vi "xiC - IMAQ - GetPRMToSave.vi"(8 "error in (no error)":errorcluster, 11 "Attributes In":T2) -> (0 "error out":errorcluster, 1 "PRM[] to Save":T1[](array[typedef]), 3 "Attributes Out":T2)   [LabVIEW 2015]
uses:
  xiCamLib/xiCam/PRM/PRM/PRM_v2.ctl
  xiC - IMAQ - Attributes.ctl
  C:/GIT/Cameras3.x/Integrations/Labview/xiLib/xiLIB_32bit/xiLIB/xiCamLib/API/x86/xiApi.NET.dll
  xiLIB_32bit/xiLIB/xiCamLib/API/x86/xiApi.NET.dll
  xiC - IMAQ - TreeDisplayType.ctl
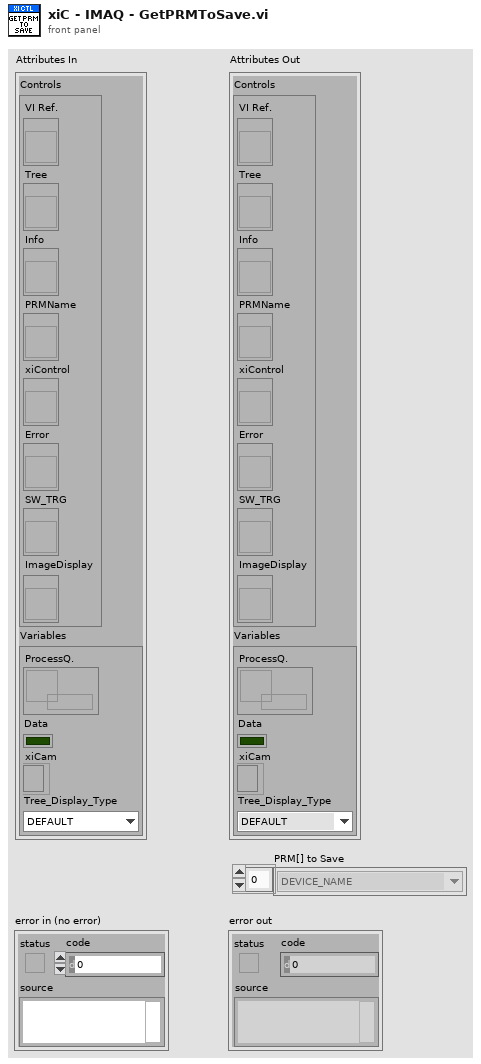
[diagram p1: front panel]
types:
  T1 = typedef "PRM_v2.ctl" = enum16{"ACQ_BUFFER_SIZE", "ACQ_FRAME_BURST_COUNT", "ACQ_TIMING_MODE", "ACQ_TRANSPORT_BUFFER_SIZE", "AE_MAX_LIMIT", "AEAG", "AEAG_LEVEL", "API_VERSION", "AG_MAX_LIMIT", "APPLY_CMS", "AUTO_BANDWIDTH_CALCULATION", "AUTO_WB", "AVAILABLE_BANDWIDTH", "AVAILABLE_BANDWIDTH_MAX", "AVAILABLE_BANDWIDTH_MIN", "BPC", "BUFFER_POLICY", "BUFFERS_QUEUE_SIZE", "CC_MATRIX_00", "CC_MATRIX_01", "CC_MATRIX_02", "CC_MATRIX_03", "CC_MATRIX_10", "CC_MATRIX_11", "CC_MATRIX_12", "CC_MATRIX_13", "CC_MATRIX_20", "CC_MATRIX_21", "CC_MATRIX_22", "CC_MATRIX_23", "CC_MATRIX_30", "CC_MATRIX_31", "CC_MATRIX_32", "CC_MATRIX_33", "CHIP_TEMP", "CMS", "COLOR_FILTER_ARRAY", "COOLING", "DEBOUNCE_EN", "DEBOUNCE_POL", "DEBOUNCE_T0", "DEBOUNCE_T1", "DEBUG_LEVEL", "DEFAULT_CC_MATRIX", "DEVICE_INSTANCE_PATH", "DEVICE_MODEL_ID", "DEVICE_NAME", "DEVICE_SN", "DEVICE_TYPE", "DEVICE_USER_ID", "DOWNSAMPLING", "DOWNSAMPLING_MAX", "DOWNSAMPLING_MIN", "DOWNSAMPLING_TYPE", "DRV_VERSION", "EXP_PRIORITY", "EXPOSURE", "EXPOSURE_DIRECT_UPDATE", "EXPOSURE_MAX", "EXPOSURE_MIN", "FFS_FILE_NAME", "FPGA1_VERSION", "FRAMERATE", "FRAMERATE_MAX", "FRAMERATE_MIN", "FREE_FFS_SIZE", "GAIN", "GAIN_DIRECT_UPDATE", "GAIN_MAX", "GAIN_MIN", "GAMMAC", "GAMMAY", "GPI_LEVEL", "GPI_MODE", "GPI_SELECTOR", "GPI_SELECTOR_MAX", "GPI_SELECTOR_MIN", "GPO_MODE", "GPO_SELECTOR", "GPO_SELECTOR_MAX", "GPO_SELECTOR_MIN", "HDR", "HDR_T1", "HDR_T2", "HEIGHT", "HEIGHT_MAX", "HEIGHT_MIN", "HOUSE_TEMP", "IMAGE_DATA_FORMAT", "IMAGE_IS_COLOR", "INPUT_CMS_PROFILE", "IS_COOLED", "IS_DEVICE_EXIST", "KNEEPOINT1", "KNEEPOINT2", "LED_MODE", "LED_SELECTOR", "LED_SELECTOR_MAX", "LED_SELECTOR_MIN", "LIMIT_BANDWIDTH", "LIMIT_BANDWIDTH_MAX", "LIMIT_BANDWIDTH_MIN", "LUT_EN", "LUT_INDEX", "LUT_INDEX_MAX", "LUT_INDEX_MIN", "LUT_VALUE", "LUT_VALUE_MAX", "LUT_VALUE_MIN", "MANUAL_WB", "MCU1_VERSION", "MCU2_VERSION", "OFFSET_X", "OFFSET_X_MAX", "OFFSET_X_MIN", "OFFSET_Y", "OFFSET_Y_MAX", "OFFSET_Y_MIN", "OUTPUT_CMS_PROFILE", "OUTPUT_DATA_BIT_DEPTH", "OUTPUT_DATA_PACKING", "READ_FILE_FFS", "RECENT_FRAME", "SENSOR_DATA_BIT_DEPTH", "SENSOR_MODE", "SENSOR_TAPS", "SHARPNESS", "SHUTTER_TYPE", "TARGET_TEMP", "TRG_DELAY", "TRG_SELECTOR", "TRG_SOFTWARE", "TRG_SOURCE", "USED_FFS_SIZE", "WB_KB", "WB_KG", "WB_KR", "WIDTH", "WIDTH_MAX", "WIDTH_MIN", "WRITE_FILE_FFS", "ACQ_BUFFER_SIZE_UNIT", "ACQ_TRANSPORT_BUFFER_COMMIT", "AEAG_ROI_HEIGHT", "AEAG_ROI_OFFSET_X", "AEAG_ROU_OFFSET_Y", "AEAG_ROI_WIDTH", "API_CONTEXT_LIST", "BINNING_HORIZONTAL", "BINNING_SELECTOR", "BINNING_VERTICAL", "COLUMN_FPN_CORRECTION", "COUNTER_SELECTOR", "COUNTER_VALUE", "DECIMATION_HORIZONTAL", "DECIMATION_SELECTOR", "DECIMATION_VERTICAL", "DEVICE_ID", "DEVICE_LOCATION_PATH", "DEVICE_MANIFEST", "DEVICE_RESET", "DEVICE_SENS_SN", "EXPOSURE_BURST_COUNT", "FFS_ACCESS_KEY", "GAIN_SELECTOR", "HW_REVISION", "IMAGE_BLACK_LEVEL", "IMAGE_DATA_BIT_DEPTH", "IMAGE_DATA_FORMAT_RGB32_ALPHA", "IMAGE_PAYLOAD_SIZE", "LENS_APERTURE_VALUE", "LENS_FEATURE", "LENS_FEATURE_SELECTOR", "LENS_FOCAL_LENGTH", "LENS_FOCUS_DISTANCE", "LENS_FOCUS_MOVE", "LENS_FOCUS_MOVEMENT_VALUE", "LENS_MODE", "OUTPUT_DATA_PACKING_TYPE", "SENSOR_CLOCK_FREQ_HZ", "SENSOR_CLOCK_FREQ_INDEX", "SENSOR_FEATURE_SELECTOR", "SENSOR_FEATURE_VALUE", "SENSOR_OUTPUT_CHANNEL_COUNT", "TRANSPORT_PIXEL_FORMAT", "TS_RST_MODE", "TS_RST_SOURCE"}
  T2 = typedef "xiC - IMAQ - Attributes.ctl" = cluster{"Controls":cluster{"VI Ref.":refnum<vi>, "Tree":refnum<vi>, "Info":refnum<vi>, "PRMName":refnum<vi>, "xiControl":refnum<vi>, "Error":refnum<vi>, "SW_TRG":refnum<vi>, "ImageDisplay":refnum<vi>}, "Variables":cluster{"ProcessQ.":refnum<queue>, "Data":bool, "xiCam":refnum<k24>, "Tree_Display_Type":T3}}
  T3 = typedef "xiC - IMAQ - TreeDisplayType.ctl" = enum16{"DEFAULT", "HIDE_MAX_MIN"}
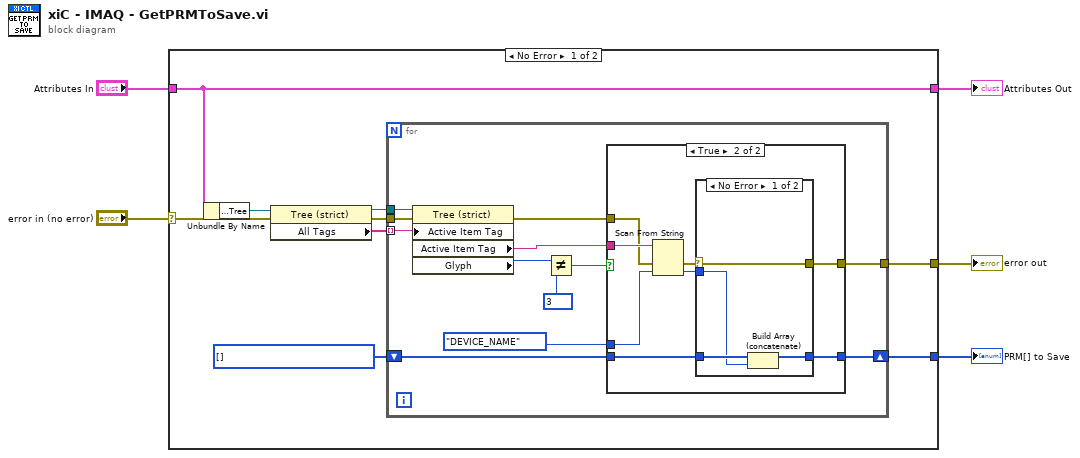
[diagram p0: block diagram]
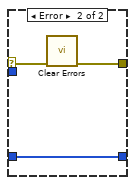
[diagram p3: hidden frame]
diagram:
  n1 = case shown="No Error" "error in (no error)" {
    selector: "error in (no error)" -> [w12 w45]
    tunnel: [w7 w45] -> w4
    tunnel: "Attributes In" -> [w13 w44]
    tunnel: [w13 w44] -> w2
    tunnel: [w6 _] -> w1
    frame No Error {
      w8 = T1[] [] items=["ACQ_BUFFER_SIZE", "ACQ_FRAME_BURST_COUNT", "ACQ_TIMING_MODE", "ACQ_TRANSPORT_BUFFER_SIZE", "AE_MAX_LIMIT", "AEAG", "AEAG_LEVEL", "API_VERSION", "AG_MAX_LIMIT", "APPLY_CMS", "AUTO_BANDWIDTH_CALCULATION", "AUTO_WB", "AVAILABLE_BANDWIDTH", "AVAILABLE_BANDWIDTH_MAX", "AVAILABLE_BANDWIDTH_MIN", "BPC", "BUFFER_POLICY", "BUFFERS_QUEUE_SIZE", "CC_MATRIX_00", "CC_MATRIX_01", "CC_MATRIX_02", "CC_MATRIX_03", "CC_MATRIX_10", "CC_MATRIX_11", "CC_MATRIX_12", "CC_MATRIX_13", "CC_MATRIX_20", "CC_MATRIX_21", "CC_MATRIX_22", "CC_MATRIX_23", "CC_MATRIX_30", "CC_MATRIX_31", "CC_MATRIX_32", "CC_MATRIX_33", "CHIP_TEMP", "CMS", "COLOR_FILTER_ARRAY", "COOLING", "DEBOUNCE_EN", "DEBOUNCE_POL", "DEBOUNCE_T0", "DEBOUNCE_T1", "DEBUG_LEVEL", "DEFAULT_CC_MATRIX", "DEVICE_INSTANCE_PATH", "DEVICE_MODEL_ID", "DEVICE_NAME", "DEVICE_SN", "DEVICE_TYPE", "DEVICE_USER_ID", "DOWNSAMPLING", "DOWNSAMPLING_MAX", "DOWNSAMPLING_MIN", "DOWNSAMPLING_TYPE", "DRV_VERSION", "EXP_PRIORITY", "EXPOSURE", "EXPOSURE_DIRECT_UPDATE", "EXPOSURE_MAX", "EXPOSURE_MIN", "FFS_FILE_NAME", "FPGA1_VERSION", "FRAMERATE", "FRAMERATE_MAX", "FRAMERATE_MIN", "FREE_FFS_SIZE", "GAIN", "GAIN_DIRECT_UPDATE", "GAIN_MAX", "GAIN_MIN", "GAMMAC", "GAMMAY", "GPI_LEVEL", "GPI_MODE", "GPI_SELECTOR", "GPI_SELECTOR_MAX", "GPI_SELECTOR_MIN", "GPO_MODE", "GPO_SELECTOR", "GPO_SELECTOR_MAX", "GPO_SELECTOR_MIN", "HDR", "HDR_T1", "HDR_T2", "HEIGHT", "HEIGHT_MAX", "HEIGHT_MIN", "HOUSE_TEMP", "IMAGE_DATA_FORMAT", "IMAGE_IS_COLOR", "INPUT_CMS_PROFILE", "IS_COOLED", "IS_DEVICE_EXIST", "KNEEPOINT1", "KNEEPOINT2", "LED_MODE", "LED_SELECTOR", "LED_SELECTOR_MAX", "LED_SELECTOR_MIN", "LIMIT_BANDWIDTH", "LIMIT_BANDWIDTH_MAX", "LIMIT_BANDWIDTH_MIN", "LUT_EN", "LUT_INDEX", "LUT_INDEX_MAX", "LUT_INDEX_MIN", "LUT_VALUE", "LUT_VALUE_MAX", "LUT_VALUE_MIN", "MANUAL_WB", "MCU1_VERSION", "MCU2_VERSION", "OFFSET_X", "OFFSET_X_MAX", "OFFSET_X_MIN", "OFFSET_Y", "OFFSET_Y_MAX", "OFFSET_Y_MIN", "OUTPUT_CMS_PROFILE", "OUTPUT_DATA_BIT_DEPTH", "OUTPUT_DATA_PACKING", "READ_FILE_FFS", "RECENT_FRAME", "SENSOR_DATA_BIT_DEPTH", "SENSOR_MODE", "SENSOR_TAPS", "SHARPNESS", "SHUTTER_TYPE", "TARGET_TEMP", "TRG_DELAY", "TRG_SELECTOR", "TRG_SOFTWARE", "TRG_SOURCE", "USED_FFS_SIZE", "WB_KB", "WB_KG", "WB_KR", "WIDTH", "WIDTH_MAX", "WIDTH_MIN", "WRITE_FILE_FFS", "ACQ_BUFFER_SIZE_UNIT", "ACQ_TRANSPORT_BUFFER_COMMIT", "AEAG_ROI_HEIGHT", "AEAG_ROI_OFFSET_X", "AEAG_ROU_OFFSET_Y", "AEAG_ROI_WIDTH", "API_CONTEXT_LIST", "BINNING_HORIZONTAL", "BINNING_SELECTOR", "BINNING_VERTICAL", "COLUMN_FPN_CORRECTION", "COUNTER_SELECTOR", "COUNTER_VALUE", "DECIMATION_HORIZONTAL", "DECIMATION_SELECTOR", "DECIMATION_VERTICAL", "DEVICE_ID", "DEVICE_LOCATION_PATH", "DEVICE_MANIFEST", "DEVICE_RESET", "DEVICE_SENS_SN", "EXPOSURE_BURST_COUNT", "FFS_ACCESS_KEY", "GAIN_SELECTOR", "HW_REVISION", "IMAGE_BLACK_LEVEL", "IMAGE_DATA_BIT_DEPTH", "IMAGE_DATA_FORMAT_RGB32_ALPHA", "IMAGE_PAYLOAD_SIZE", "LENS_APERTURE_VALUE", "LENS_FEATURE", "LENS_FEATURE_SELECTOR", "LENS_FOCAL_LENGTH", "LENS_FOCUS_DISTANCE", "LENS_FOCUS_MOVE", "LENS_FOCUS_MOVEMENT_VALUE", "LENS_MODE", "OUTPUT_DATA_PACKING_TYPE", "SENSOR_CLOCK_FREQ_HZ", "SENSOR_CLOCK_FREQ_INDEX", "SENSOR_FEATURE_SELECTOR", "SENSOR_FEATURE_VALUE", "SENSOR_OUTPUT_CHANNEL_COUNT", "TRANSPORT_PIXEL_FORMAT", "TS_RST_MODE", "TS_RST_SOURCE"]
      n2 = Unbundle By Name(w13) -> ("Controls.Tree"=w14:refnum<vi>)
      n3 = property class="Tree (strict)"(reference=w14, error in=w12) -> (reference out=w11:refnum<vi>, error out=w10:errorcluster, "All Tags"=w9:string[])
      n4 = for {
        tunnel: w11 -> [w26]
        tunnel: w10 -> [w24]
        tunnel: w9 -> [w25] mode=indexing
        tunnel: [w19] -> w7
        shift-right: [w17] -> w6
        shift-left: w8 -> [w18]
        n5 = property class="Tree (strict)"(reference=w26, error in=w24, "Active Item Tag"=w25) -> (error out=w21:errorcluster, "Active Item Tag"=w22:string, "Glyph"=w16:i32)  [unwired: 1 out]
        n6 = Not Equal?(x=w16, y=3) -> (x != y?=w15:bool)
        n7 = case shown="True" w15 {
          tunnel: w22 -> [_ w36]
          tunnel: w21 -> [w28 w35]
          tunnel: PRM_v2."DEVICE_NAME" ("PRM") -> [_ w34]
          tunnel: [w28 w32] -> w19
          tunnel: w18 -> [w27 w30]
          tunnel: [w27 w29] -> w17
          frame False {
          }
          frame True {
            n8 = Scan From String(input string=w36, error in=w35, default 1=w34) -> (error out=w33:errorcluster, output 1=w31:T1)  [unwired: 2 in, 2 out]
            n9 = case shown="No Error" w33 {
              selector: w33 -> [w40 w43]
              tunnel: [w40 w42] -> w32
              tunnel: w31 -> [w38 _]
              tunnel: w30 -> [w39 w41]
              tunnel: [w37 w41] -> w29
              frame No Error {
                n10 = Build Array (concatenate)(w39, w38) -> (w37:T1[])
              }
              frame Error {
                n11 = call <vilib>:"Clear Errors.vi"("error in (no error)"=w43) -> ("error out"=w42:errorcluster)  [unwired: 5 in, 1 out]
              }
            }
          }
        }
      }
    }
    frame Error {
    }
  }
  "error out" <- w4
  "Attributes Out" <- w2
  "PRM[] to Save" <- w1
